vi "read.vi"(8 "error in (no error)":errorcluster, 10 "ElectrometerController in":refnum<class "ElectrometerController.lvclass">, 11 "UntilIntensityReading in":refnum<class "UntilIntensityReading.lvclass">) -> (0 "error out":errorcluster, 1 "lastMeasure":dbl, 2 "ElectrometerController out":refnum<class "ElectrometerController.lvclass">, 3 "UntilIntensityReading out":refnum<class "UntilIntensityReading.lvclass">, 4 "newValue":bool)   [LabVIEW 2016, in "UntilIntensityReading.lvclass"]
uses:
  UntilIntensityReading.lvclass
  ElectrometerController/ElectrometerController.lvclass
  State.lvclass
  Electrometer.lvclass
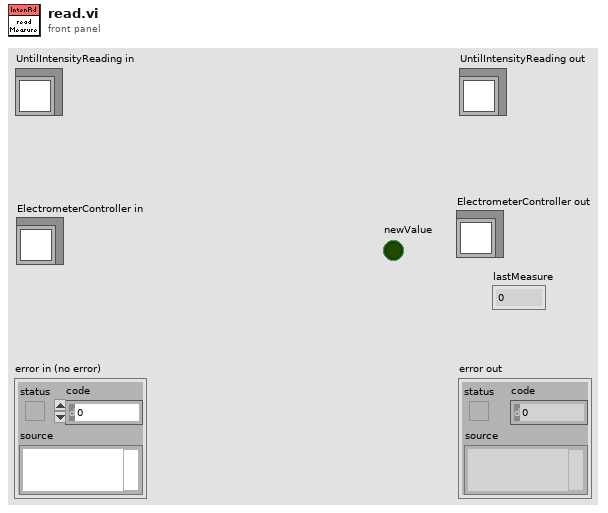
[diagram p1: front panel]
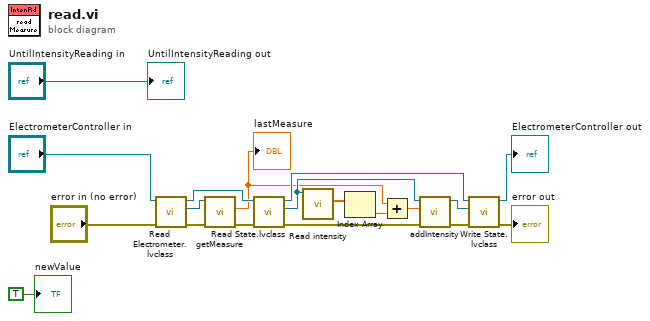
[diagram p0: block diagram]
diagram:
  n1 = call-dynamic "Read Electrometer.lvclass.vi"("error in (no error)"="error in (no error)", "ElectrometerController in"="ElectrometerController in") -> ("error out"=w15:errorcluster, "Electrometer.lvclass"=w16:refnum<class "Electrometer.lvclass">, "ElectrometerController out"=w14:refnum<class "ElectrometerController.lvclass">)  [unwired: 7 in]
  n2 = call "getMeasure.vi"("error in (no error)"=w15, "Electrometer in"=w16) -> ("error out"=w13:errorcluster, "Measure"=w2:dbl)  [unwired: 7 in, 1 out]
  "lastMeasure" <- w2
  n3 = call-dynamic "Read State.lvclass.vi"("error in (no error)"=w13, "ElectrometerController in"=w14) -> ("error out"=w12:errorcluster, "State.lvclass"=w5:refnum<class "State.lvclass">, "ElectrometerController out"=w9:refnum<class "ElectrometerController.lvclass">)  [unwired: 7 in]
  n4 = call-dynamic "Read intensity.vi"("State in"=w5) -> ("intensity"=w4:dbl[])  [unwired: 8 in, 2 out]
  n5 = Index Array(array=w4) -> (element=w3:dbl)  [unwired: 1 in]
  n6 = Add(x=w2, y=w3) -> (x+y=w1:dbl)
  n7 = call-dynamic "addIntensity.vi"("error in (no error)"=w12, "lastMeasure"=w1, "State in"=w5) -> ("error out"=w11:errorcluster, "State out"=w10:refnum<class "State.lvclass">)  [unwired: 7 in]
  n8 = call-dynamic "Write State.lvclass.vi"("error in (no error)"=w11, "State.lvclass"=w10, "ElectrometerController in"=w9) -> ("error out"=→"error out":errorcluster, "ElectrometerController out"=→"ElectrometerController out":refnum<class "ElectrometerController.lvclass">)  [unwired: 7 in]
  "UntilIntensityReading out" <- "UntilIntensityReading in"
  "newValue" <- TRUE ("newValue")
